vi "Dashboard Main.vi"() -> ()   [LabVIEW 2023]
uses:
  52f2dcef-b32f-41dc-9262-467f65fbdc6c.vi
  <vilib>/Rock Robotics/Network Tables/NT Write String Array.vi
  <vilib>/Rock Robotics/WPI/Dashboard/WPI_DashboardLogging Global.vi
  <vilib>/Rock Robotics/Network Tables/NT Write Boolean.vi
panel:
  in  "Camera Settings Right":T1={"Frame Rate"=30, "Compression"=30, "Size"=1, "DB Camera Config"=FALSE} {"Frame Rate" scale=1.0..30.0; "Compression" scale=100.0..-1.0; "Size" items=["640x480", "320x240", "160x120"]}
  in  "Camera Name Right":string(combo)="No Camera Selection"
  out "NT Connection":bool
  in  "Camera Settings":T1={"Frame Rate"=30, "Compression"=30, "Size"=1, "DB Camera Config"=FALSE} {"Frame Rate" scale=1.0..30.0; "Compression" scale=100.0..-1.0; "Size" items=["640x480", "320x240", "160x120"]}
  in  "Camera Name":string(combo)="No Camera Selection"
  in  "TCP":refnum<k5>
  in  "Rec Mode":enum32{"Stop", "Record", "Playback"}(radio)
  out "Robot IP":string
  out "Image Message":string="Timeout in Camera Communications"
  in  "Dashboard Tab":T2(tab)
  out "Bottom Left Flywheel":dbl
  out "Top Left Flywheel":dbl
  in  "Battery Used":string
  in  "Auto Delay?":bool
  in  "Delay Time (s)":dbl
  out "Climb 2":dbl
  in  "Aquitaine File":string
  in  "Climb Arm Reset":bool
  out "Climb 1":dbl
  out "Bottom Right Flywheel":dbl
  out "Top Right Flywheel":dbl
  in  "Shooter Hood Reset":bool
  in  "Auto Calibrate":bool=TRUE
  in  "Robot Selector":u16(ring) items=["2468 Competition", "2468 Practice"]
  in  "Manual Paths":string[](array[string])
  in  "Max Rotation":dbl=270.0
  in  "Max Translation":dbl=19.0
  in  "Deadband":dbl=0.05
  in  "Auto Selector":T3(ring)
  out "IMU":dbl(knob) scale=-180.0..180.0
  in  "Select Auto":string(combo)="Select Autonomous ..."
  out "Mode":T4(ring)=enum."Auto Disabled"
  out "Camera Perf":cluster{"Bandwidth (Mbps)":dbl, "FPS":dbl}
  out "Shooter Hood":dbl
  out "Camera Perf 2":string
  out "Auto Picture":picture
  in  "Amp Scale":dbl=0.97
  out "Shooter Hood":dbl
  out "Distance from Speaker":dbl
  out "Trap Auto Align":bool
  out "Camera Image Right":T5(plugin-control)
  out "Speaker Auto Align":bool
  out "Field Centric":bool
  out "Camera Image":T5(plugin-control)
  out "Current Shot":T6(ring)
  out "In Range?":bool
  out "Tree":string(tree)
  # "HW"
  # "HW"
  # "IMU"
  # "SWERVE"
  # "AUTONOMOUS"
  # "CONFIGS"
  # "FEEDBACK"
  # "INTAKE VIEW"
  # "SHOOTER VIEW"
  # "FIELD CENTRIC"
  # "SPEAKER AA"
  # "TRAP AA"
  # "CAN ERROR"
  # "SENSOR FAULT"
  # "GATE DRIVER"
  # "No POWER"
  # "FuLL FORWARD"
  # "FuLL REVERSE"
  # "BRUSHED BRAKE"
  # "BRUSHED COAST"
  # "BRUSHLESS BRAKE"
  # "BRUSHLESS COAST"
  # "RECOVERY MODE/OFF"
  # "https://cdn8.bigcommerce.com/s-t3eo8vwp22/product_images/uploaded_images/fault-no-12v.gif"
  # "PIGEON 2"
  # "DAMAGED HARDWARE"
  # "BOOTLOADER"
  # "CAN FAULT"
  # "ROBOT DISABLED"
  # "ROBOT ENABLED"
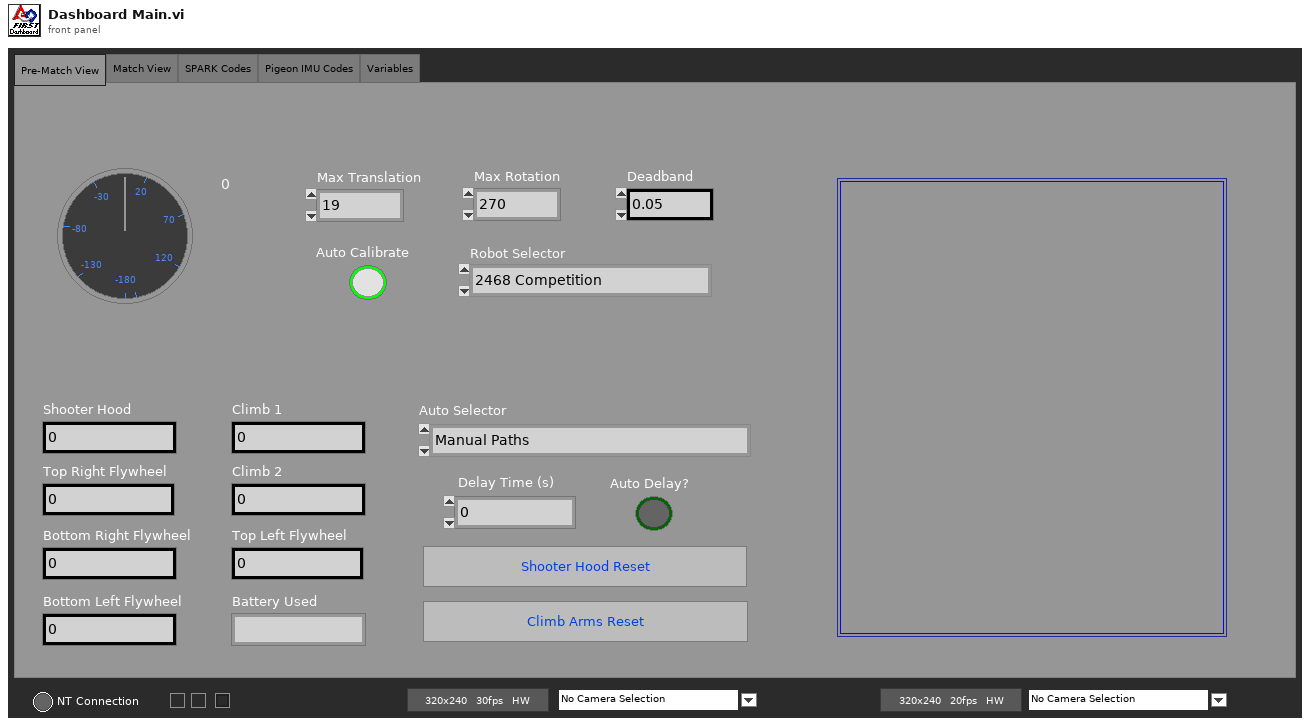
[diagram p1: front panel]
types:
  T1 = cluster{"Frame Rate":i32, "Compression":i32, "Size":u16, "DB Camera Config":bool}
  T2 = enum32{"Pre-Match View", "Match View", "SPARK Codes", "Pigeon IMU Codes", "Variables"}
  T3 = enum16{"Manual Paths", "Center - 5 Note (Line + 3rd)", "Center - 4 Note (Line + Sprint)", "Amp RED - 5 Note (1 then 3)", "Amp BLUE - 5 Note (1 then 3)", "Source RED - 3 Note (5, 4, Sprint)", "Source BLUE - 3 Note (5, 4, Sprint)", "Source RED - 3 Note (4, 5, Sprint)", "Source BLUE - 3 Note (4, 5, Sprint)", "Center - 5 Note (3, 2, 4)"}
  T4 = enum8{"Tele-Op Disabled", "Tele-Op Enabled", "Auto Disabled", "Auto Enabled", "Test Disabled", "Test Enabled", "Disconnected", "No Code", "E-Stop"}
  T5 = typedef "IMAQ Image.ctl" = refnum<image>
  T6 = enum32{"Soft Lob", "Amp", "Subwoofer", "Long Lob", "Idle", "Zero", "Trap", "Interpolation"}
  T7 = cluster{"Save Path":path, "Interval (s)":dbl, "Keep":i32}
  T8 = typedef "Image Type" = u32
  T9 = enum32{"Pre-Match View", "Match View", "SparkMax Codes", "Pigeon IMU Codes", "Variables"}
  T10 = cluster{"IDs":cluster{"RPC field ID":u16, "Unique ID":u16}, "String":string}
  T11 = cluster{"Dashboard Tab":refnum<vi>, "Rec Mode":refnum<vi>, "Tree":refnum<vi>, "Camera Perf 2":refnum<vi>, "Camera Settings":refnum<vi>, "Camera Name":refnum<vi>, "Camera Image":refnum<vi>}
  T12 = cluster{"Global Rectangle":i32[], "Contours":cluster{"Contour Type":u32, "ROI Type":u32, "Points":i32[]}[]}
  T13 = cluster{"Camera Name Right":string, string, "Saved DB Images Info":cluster{"Save Path":path, "Interval (s)":dbl, "Keep":i32}}
  T14 = cluster{"Camera Name":string, string, "Saved DB Images Info":cluster{"Save Path":path, "Interval (s)":dbl, "Keep":i32}}
  T15 = cluster{"Error Strings":string, "Disable Counts":cluster{u16, u16}, "Rail Faults":cluster{u16, u16, u16}, "Robot IP":string, "DB Mode":u8, "Event Info":cluster{"Name":string, "Type":u8, "Number":u16, "Replay":u8}}
  T16 = cluster{"Storage":cluster{"Disk Free":u64, "RAM Block":u32, "RAM free":u32}, "CPU Utilization":cluster{"CPU % ISR":sgl, "CPU % Time Crit":sgl, "CPU % Timed Str":sgl, "CPU % High":sgl, "CPU % Above":sgl, "CPU % Normal":sgl, "CPU % Low":sgl}, "CAN":cluster{"% Bus Utilization":sgl, "Bus Off Cnt":u32, "TX_FIFO Full Cnt":u32, "Receive Error Cnt":u8, "Transmit Error Cnt":u8}, "HID":cluster{"HID Outputs":u32, "Rumble Low":u16, "Rumble High":u16}[]}
  T17 = cluster{"Status bits":cluster{"Test Mode":bool, "Autonomous":bool, "Enabled":bool, "Code Start":bool, "Brownout":bool, "Reserved 2":bool, "Reserved 3":bool, "E-Stop":bool}, "Code Trace":cluster{"Disabled":bool, "TeleOp":bool, "Auto":bool, "Test":bool}, "Controller Type":enum16{"unknown", "cRIO", "roboRio"}, "Code?":enum16{"unknown", "noCode", "code"}, "Battery V":dbl}
  T18 = cluster{"Control Bits":cluster{"TestMode":bool, "Autonomous":bool, "Enabled":bool, "FMS Present":bool, bool, bool, bool, "E-Stop":bool}, "Team Station ":u8, "Countdown":sgl, "Joystick Values":cluster{"Axes":dbl[], "Buttons":bool[], "POVs":i16[]}[]}
  T19 = typedef "imagedata.ctl" = cluster{"image type":i32, "image depth":i32, "image":u8[], "mask":u8[], "colors":u32[], "Rectangle":cluster{"left":i16, "top":i16, "right":i16, "bottom":i16}}
  T20 = cluster{"Operation":enum16{"Update", "Clear"}, "Color Box":u32}[]
  T21 = cluster{"Image Size":bool, "Image Type":bool, "Pixel Value":bool, "ROI Information":bool, "Zoom Factor":bool}
  T22 = cluster{"Shift":bool, "Ctrl":bool, "Alt":bool, "Cmd":bool, "Opt":bool}
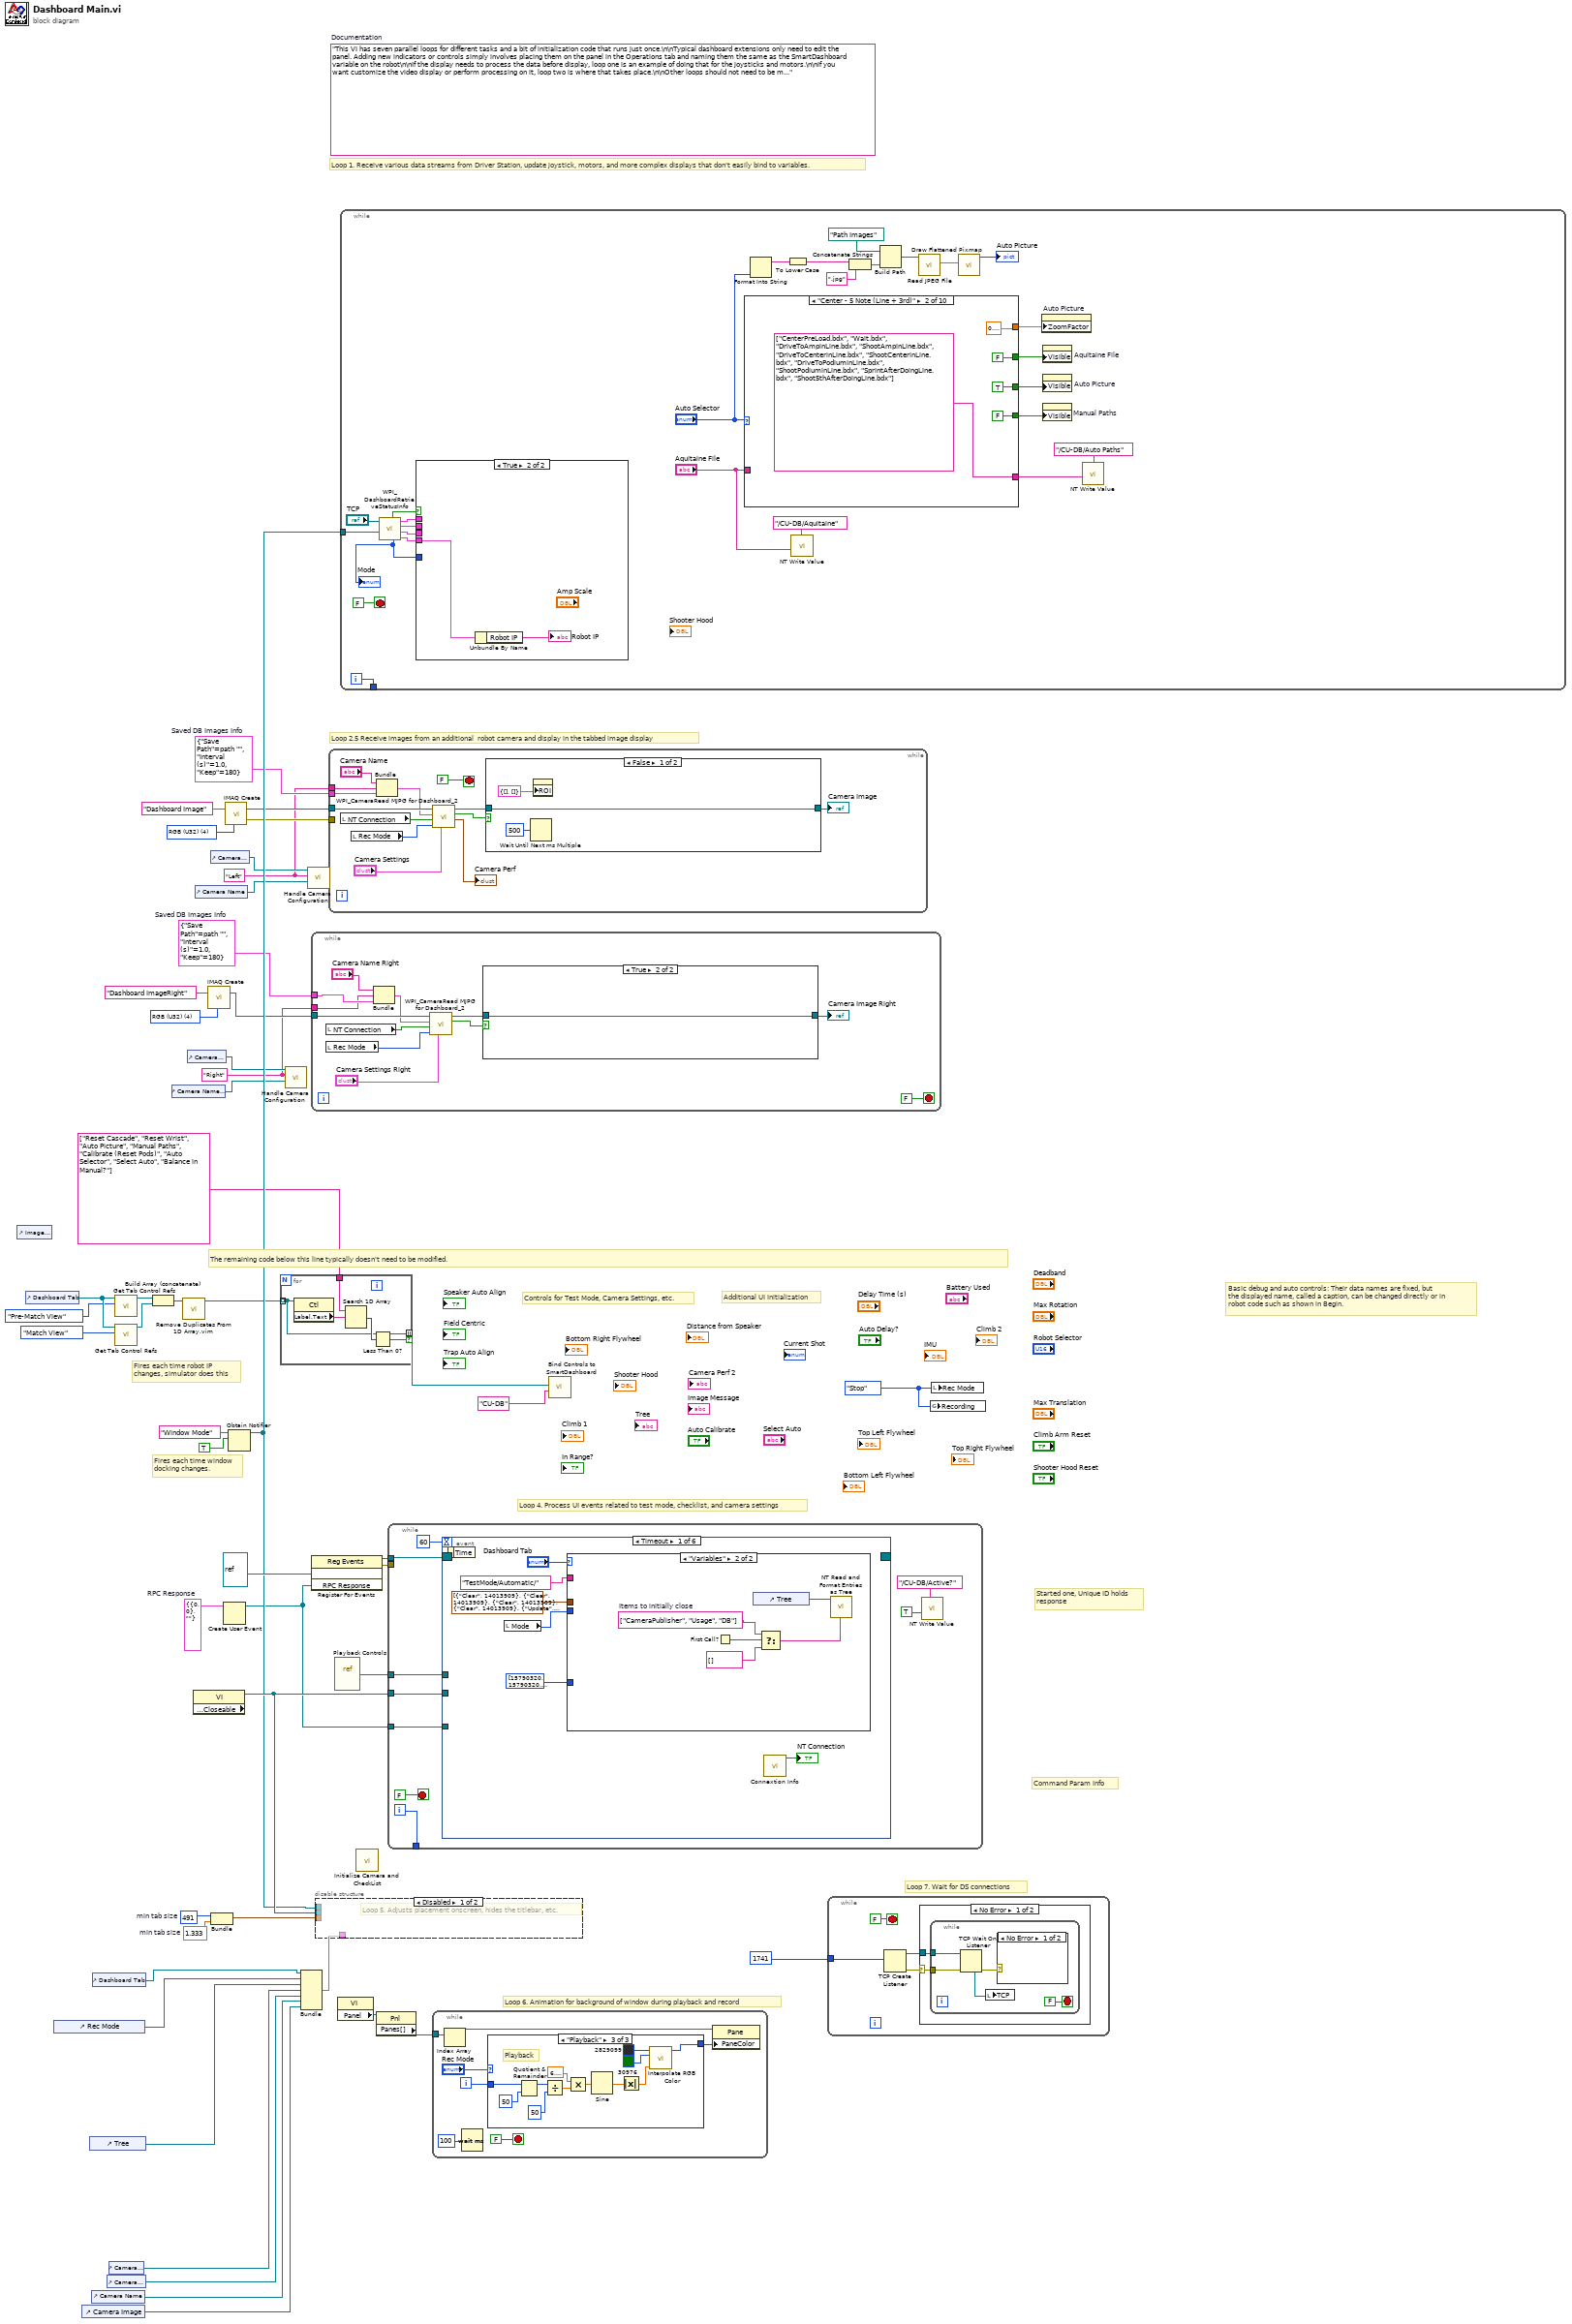
[diagram p0: block diagram]
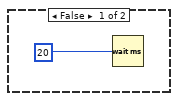
[diagram p2: hidden frame]
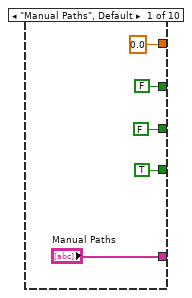
[diagram p3: hidden frame]
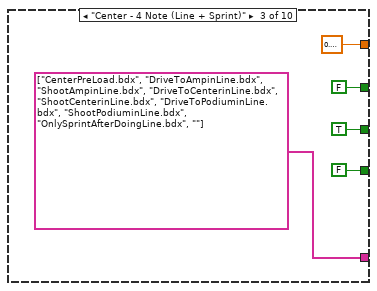
[diagram p4: hidden frame]
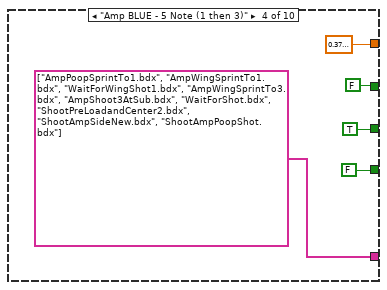
[diagram p5: hidden frame]
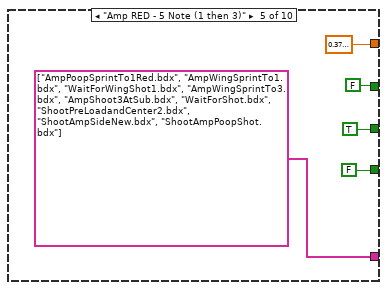
[diagram p6: hidden frame]
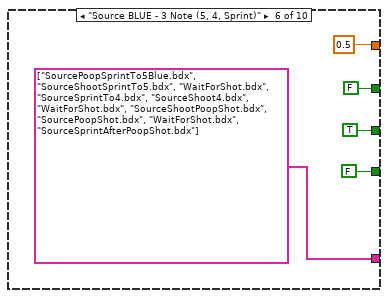
[diagram p7: hidden frame]
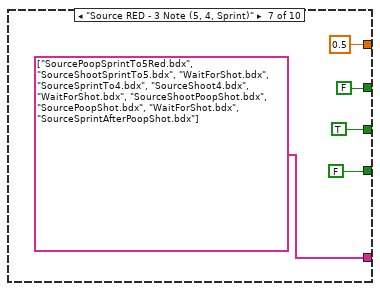
[diagram p8: hidden frame]
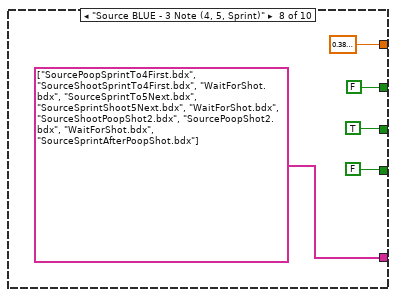
[diagram p9: hidden frame]
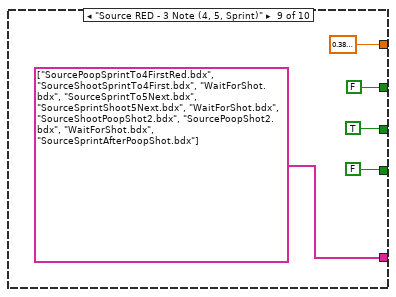
[diagram p10: hidden frame]
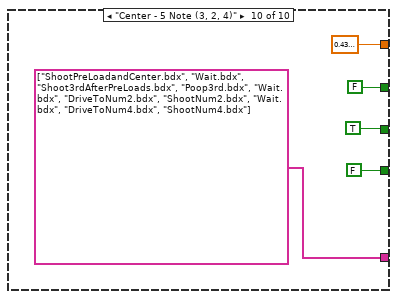
[diagram p11: hidden frame]
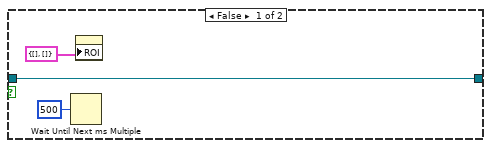
[diagram p14: hidden frame]
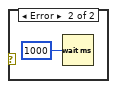
[diagram p15: hidden frame]
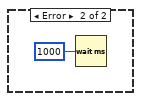
[diagram p16: hidden frame]
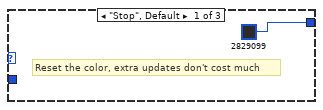
[diagram p17: hidden frame]
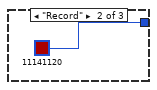
[diagram p18: hidden frame]
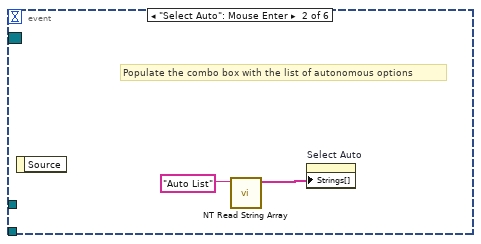
[diagram p20: hidden frame]
diagram:
  w1 = "Right"
  w6 = T7 {"Save Path"=path "", "Interval (s)"=1.0, "Keep"=180}  # Saved DB Images Info
  w8 = T8 4 items=["Grayscale (U8)", "Grayscale (I16)", "Grayscale (SGL)", "Complex (CSG)", "RGB (U32)", "HSL (U32)", "RGB (U64)"] ("Image Type")
  w24 = T7 {"Save Path"=path "", "Interval (s)"=1.0, "Keep"=180}  # Saved DB Images Info
  w5 = "Left"
  w29 = T8 4 items=["Grayscale (U8)", "Grayscale (I16)", "Grayscale (SGL)", "Complex (CSG)", "RGB (U32)", "HSL (U32)", "RGB (U64)"] ("Image Type")
  w33 = T10 {"IDs"={"RPC field ID"=0, "Unique ID"=0}, "String"=""}  # RPC Response
  w40 = 491  # min tab size
  w39 = 1.333  # min tab size
  w42 = enum32{"Stop", "Record", "Playback"}."Stop" ("Rec Mode")
  (unwired) "This VI has seven parallel loops for different tasks and a bit of initialization code that runs just once.\n\nTypical dashboard extensions only need to edit the panel. Adding new indicators or controls simply involves placing them on the panel in the Operations tab and naming them the same as the SmartDashboard variable on the robot\n\nIf the display needs to process the data before display, loop one is an example of doing that for the joysticks and motors.\n\nIf you want customize the video display or perform processing on it, loop two is where that takes place.\n\nOther loops should not need to be modified. They are pretty standard, and document the task they perform."  # Documentation
  # "Loop 2.5 Receive images from an additional  robot camera and display in the tabbed image display"
  # "Command Param Info"
  # "Started one, Unique ID holds\nresponse"
  # "Loop 7. Wait for DS connections"
  # "Basic debug and auto controls: Their data names are fixed, but\nthe displayed name, called a caption, can be changed directly or in\nrobot code such as shown in Begin."
  # "Controls for Test Mode, Camera Settings, etc."
  # "Additional UI Initialization"
  # "Loop 6. Animation for background of window during playback and record"
  # "Fires each time robot IP\nchanges, simulator does this"
  # "Fires each time window\ndocking changes."
  # "The remaining code below this line typically doesn't need to be modified."
  # "Loop 4. Process UI events related to test mode, checklist, and camera settings"
  # "Loop 1. Receive various data streams from Driver Station, update joystick, motors, and more complex displays that don't easily bind to variables."
  n1 = control-ref of="Image Message"() -> ()  [unwired: 1 out]
  n2 = control-ref of="Dashboard Tab"() -> (w22:refnum<vi>)
  n3 = control-ref of="Rec Mode"() -> (w36:refnum<vi>)
  n4 = control-ref of="Camera Image"() -> (w25:refnum<vi>)
  n5 = control-ref of="Tree"() -> (w23:refnum<vi>)
  n6 = control-ref of="Camera Name"() -> (w26:refnum<vi>)
  n7 = control-ref of="Dashboard Tab"() -> (w14:refnum<vi>)
  n8 = control-ref of="Camera Settings"() -> (w27:refnum<vi>)
  n9 = control-ref of="Camera Perf 2"() -> (w31:refnum<vi>)
  n10 = call <vilib>:"Get Tab Control Refs.vi"("Page Index"=T9."Pre-Match View" ("Dashboard Tab"), "TabControl in"=w22) -> ("ControlsOnPage"=w21:refnum<vi>[])  [unwired: 9 in]
  n11 = call <vilib>:"Get Tab Control Refs.vi"("Page Index"=T9."Match View" ("Dashboard Tab"), "TabControl in"=w22) -> ("ControlsOnPage"=w20:refnum<vi>[])  [unwired: 9 in]
  n12 = Build Array (concatenate)(w21, w20) -> (w19:refnum<vi>[])
  n13 = control-ref of="Camera Name Right"() -> (w2:refnum<vi>)
  n14 = call "Remove Duplicates From 1D Array.vim"("array"=w19) -> ("array with duplicates removed"=w16:refnum<vi>[])  [unwired: 10 in]
  n15 = control-ref of="Camera Settings Right"() -> (w3:refnum<vi>)
  n16 = property class="VI" props=["Front Panel.Closeable"]() -> (reference out=w41:refnum<vi>)  [unwired: 2 in, 2 out]
  n17 = control-ref of="Camera Name"() -> (w10:refnum<vi>)
  n18 = call "IMAQ Create"("Image Name"="Dashboard ImageRight", "Image Type"=w8) -> ("New Image"=w4:T5)  [unwired: 2 in, 2 out]
  n19 = control-ref of="Camera Settings"() -> (w11:refnum<vi>)
  n20 = Bundle("min tab size"=w40, "min tab size"=w39) -> (w38:cluster{"min tab size":i32, "min tab size":dbl})  [unwired: 1 in]
  n21 = Create User Event(user event datatype=w33) -> (user event=w32:refnum<user-event>)  [unwired: 1 in, 1 out]
  n22 = call "IMAQ Create"("Image Name"="Dashboard Image", "Image Type"=w29) -> ("New Image"=w9:T5, "error out"=w28:errorcluster)  [unwired: 2 in, 1 out]
  n23 = Obtain Notifier(name (unnamed)="Window Mode", notification data type=TRUE) -> (notifier out=w35:refnum<notifier>)  [unwired: 2 in, 2 out]
  n24 = for {
    tunnel: string[] ["Reset Cascade", "Reset Wrist", "Auto Picture", "Manual Paths", "Calibrate (Reset Pods)", "Auto Selector", "Select Auto", "Balance in Manual?"] -> [w56]
    tunnel: w16 -> [w53] mode=indexing
    tunnel: [w53] -> w15 mode=indexing if=w52
    n25 = property class="Ctl"(reference=w53) -> ("Label.Text"=w55:string)  [unwired: 1 in, 2 out]
    n26 = Search 1D Array(1D array=w56, element=w55) -> (index of element=w54:i32)  [unwired: 1 in]
    n27 = Less Than 0?(x=w54) -> (x < 0?=w52:bool)
  }
  n28 = call "Handle Camera Configuration.vi"("CameraNameRef"=w2, "Display Name"=w1, "ClusterRef"=w3) -> ()  [unwired: 9 in]
  n29 = Bundle("Dashboard Tab"=w14, "Rec Mode"=w36, "Tree"=w23, "Camera Perf 2"=w31, "Camera Settings"=w27, "Camera Name"=w26, "Camera Image"=w25) -> (w37:T11)  [unwired: 1 in]
  n30 = call "Handle Camera Configuration.vi"("CameraNameRef"=w10, "Display Name"=w5, "ClusterRef"=w11) -> ()  [unwired: 9 in]
  n31 = while {
    tunnel: w6 -> [w61]
    tunnel: w4 -> [w64]
    tunnel: w1 -> [w58]
    stop <- FALSE stop-if-true
    n32 = local read "NT Connection"() -> (w63:bool)
    n33 = local read "Rec Mode"() -> (w62:enum32{"Stop", "Record", "Playback"})
    n34 = Bundle("Camera Name Right"="Camera Name Right", w58, "Saved DB Images Info"=w61) -> (w57:T13)  [unwired: 1 in]
    n35 = call <vilib>:"WPI_CameraRead MJPG for Dashboard_2.vi"("Camera Settings"="Camera Settings Right", "Rec Mode"=w62, "NT Connection"=w63, "Capture Info"=w57, "Image in"=w64) -> ("Active"=w66:bool, "Image\\ out"=w67:T5)  [unwired: 4 in, 1 out]
    n36 = case shown="True" w66 {
      tunnel: w67 -> [w70 w72]
      tunnel: [w70 w72] -> w68
      frame False {
        n37 = Wait Until Next ms Multiple(millisecond multiple=u32 500) -> ()  [unwired: 1 out]
        n38 = property on="Camera Image" class="ImageControl"("ROI"=T12 {"Global Rectangle"=[], "Contours"=[]}) -> ()  [unwired: 2 in, 2 out]
      }
      frame True {
      }
    }
    "Camera Image Right" <- w68
  }
  n39 = register-events(refnum<vi> refnum, w32) -> (reference out=w45:refnum<event-registration>, error out=w44:errorcluster)  [unwired: 2 in]
  n40 = disable-structure shown="Disabled" {
    disable-tunnel: w41 -> [_ _]
    disable-tunnel: w38 -> [_ _]
    disable-tunnel: w37 -> [_ _]
    disable-tunnel: w35 -> [_ _]
    frame Disabled {
      # "Loop 5. Adjusts placement onscreen, hides the titlebar, etc."
    }
    frame Enabled {
    }
  }
  n41 = while {
    tunnel: w9 -> [w85]
    tunnel: w28 -> [_]
    tunnel: w24 -> [w74]
    tunnel: w5 -> [w76]
    stop <- FALSE stop-if-true
    n42 = local read "NT Connection"() -> (w75:bool)
    n43 = local read "Rec Mode"() -> (w73:enum32{"Stop", "Record", "Playback"})
    n44 = Bundle("Camera Name"="Camera Name", w76, "Saved DB Images Info"=w74) -> (w79:T14)  [unwired: 1 in]
    n45 = call <vilib>:"WPI_CameraRead MJPG for Dashboard_2.vi"("Camera Settings"="Camera Settings", "Rec Mode"=w73, "NT Connection"=w75, "Capture Info"=w79, "Image in"=w85) -> ("perf info"=→"Camera Perf":cluster{"Bandwidth (Mbps)":dbl, "fps":dbl}, "Active"=w81:bool, "Image\\ out"=w83:T5)  [unwired: 4 in]
    n46 = case shown="False" w81 {
      tunnel: w83 -> [w87 w89]
      tunnel: [w87 w89] -> w80
      frame False {
        n47 = Wait Until Next ms Multiple(millisecond multiple=u32 500) -> ()  [unwired: 1 out]
        n48 = property on="Camera Image" class="ImageControl"("ROI"=T12 {"Global Rectangle"=[], "Contours"=[]}) -> ()  [unwired: 2 in, 2 out]
      }
      frame True {
      }
    }
    "Camera Image" <- w80
  }
  n49 = vi-ref "Playback Controls.vi"() -> (w46:refnum<vi>)
  n50 = property class="VI"() -> ("Panel"=w48:refnum<vi>)  [unwired: 2 in, 2 out]
  n51 = while {
    tunnel: [w115] -> _
    tunnel: w35 -> [w108]
    i -> [w115]
    stop <- FALSE stop-if-true
    n52 = call <vilib>:"WPI_DashboardRetrieveStatusInfo.vi"("Window Mode Notifier"=w108, "TCP Cnx"="TCP") -> ("Power and Errors"=w110:T15, "Robot Metrics"=w113:T16, "Status Info"=w114:T17, "Control Info"=w111:T18, "Robot Mode"=w91:T4, "Process?"=w112:bool)  [unwired: 4 in]
    "Mode" <- w91
    n53 = case shown="True" w112 {
      tunnel: w114 -> [_ _]
      tunnel: w113 -> [_ _]
      tunnel: w111 -> [_ _]
      tunnel: w110 -> [_ w119]
      tunnel: w91 -> [_ _]
      frame False {
        n54 = Wait (ms)(milliseconds to wait=u32 20) -> ()  [unwired: 1 out]
      }
      frame True {
        n55 = Unbundle By Name(w119) -> ("Robot IP"=→"Robot IP":string)
      }
    }
    n56 = case shown="\"Center - 5 Note (Line + 3rd)\"" "Auto Selector" {
      tunnel: ["Manual Paths" string[] ["CenterPreLoad.bdx", "Wait.bdx", "DriveToAmpinLine.bdx", "ShootAmpinLine.bdx", "DriveToCenterinLine.bdx", "ShootCenterinLine.bdx", "DriveToPodiuminLine.bdx", "ShootPodiuminLine.bdx", "SprintAfterDoingLine.bdx", "Shoot5thAfterDoingLine.bdx"] ("Manual Paths") string[] ["CenterPreLoad.bdx", "DriveToAmpinLine.bdx", "ShootAmpinLine.bdx", "DriveToCenterinLine.bdx", "ShootCenterinLine.bdx", "DriveToPodiuminLine.bdx", "ShootPodiuminLine.bdx", "OnlySprintAfterDoingLine.bdx", ""] ("Manual Paths") string[] ["AmpPoopSprintTo1.bdx", "AmpWingSprintTo1.bdx", "WaitForWingShot1.bdx", "AmpWingSprintTo3.bdx", "AmpShoot3AtSub.bdx", "WaitForShot.bdx", "ShootPreLoadandCenter2.bdx", "ShootAmpSideNew.bdx", "ShootAmpPoopShot.bdx"] ("Manual Paths") string[] ["AmpPoopSprintTo1Red.bdx", "AmpWingSprintTo1.bdx", "WaitForWingShot1.bdx", "AmpWingSprintTo3.bdx", "AmpShoot3AtSub.bdx", "WaitForShot.bdx", "ShootPreLoadandCenter2.bdx", "ShootAmpSideNew.bdx", "ShootAmpPoopShot.bdx"] ("Manual Paths") string[] ["SourcePoopSprintTo5Blue.bdx", "SourceShootSprintTo5.bdx", "WaitForShot.bdx", "SourceSprintTo4.bdx", "SourceShoot4.bdx", "WaitForShot.bdx", "SourceShootPoopShot.bdx", "SourcePoopShot.bdx", "WaitForShot.bdx", "SourceSprintAfterPoopShot.bdx"] ("Manual Paths") string[] ["SourcePoopSprintTo5Red.bdx", "SourceShootSprintTo5.bdx", "WaitForShot.bdx", "SourceSprintTo4.bdx", "SourceShoot4.bdx", "WaitForShot.bdx", "SourceShootPoopShot.bdx", "SourcePoopShot.bdx", "WaitForShot.bdx", "SourceSprintAfterPoopShot.bdx"] ("Manual Paths") string[] ["SourcePoopSprintTo4First.bdx", "SourceShootSprintTo4First.bdx", "WaitForShot.bdx", "SourceSprintTo5Next.bdx", "SourceSprintShoot5Next.bdx", "WaitForShot.bdx", "SourceShootPoopShot2.bdx", "SourcePoopShot2.bdx", "WaitForShot.bdx", "SourceSprintAfterPoopShot.bdx"] ("Manual Paths") string[] ["SourcePoopSprintTo4FirstRed.bdx", "SourceShootSprintTo4First.bdx", "WaitForShot.bdx", "SourceSprintTo5Next.bdx", "SourceSprintShoot5Next.bdx", "WaitForShot.bdx", "SourceShootPoopShot2.bdx", "SourcePoopShot2.bdx", "WaitForShot.bdx", "SourceSprintAfterPoopShot.bdx"] ("Manual Paths") string[] ["ShootPreLoadandCenter.bdx", "Wait.bdx", "Shoot3rdAfterPreLoads.bdx", "Poop3rd.bdx", "Wait.bdx", "DriveToNum2.bdx", "ShootNum2.bdx", "Wait.bdx", "DriveToNum4.bdx", "ShootNum4.bdx"] ("Manual Paths")] -> w107
      tunnel: [FALSE ("Visible") TRUE ("Visible") TRUE ("Visible") TRUE ("Visible") TRUE ("Visible") TRUE ("Visible") TRUE ("Visible") TRUE ("Visible") TRUE ("Visible") TRUE ("Visible")] -> w106
      tunnel: [TRUE ("Visible") FALSE ("Visible") FALSE ("Visible") FALSE ("Visible") FALSE ("Visible") FALSE ("Visible") FALSE ("Visible") FALSE ("Visible") FALSE ("Visible") FALSE ("Visible")] -> w93
      tunnel: [FALSE ("Visible") FALSE ("Visible") FALSE ("Visible") FALSE ("Visible") FALSE ("Visible") FALSE ("Visible") FALSE ("Visible") FALSE ("Visible") FALSE ("Visible") FALSE ("Visible")] -> w103
      tunnel: "Aquitaine File" -> [_ _ _ _ _ _ _ _ _ _]
      tunnel: [sgl 0.0 ("Zoom Factor") sgl 0.4 ("Zoom Factor") sgl 0.4 ("Zoom Factor") sgl 0.37 ("Zoom Factor") sgl 0.37 ("Zoom Factor") sgl 0.5 ("Zoom Factor") sgl 0.5 ("Zoom Factor") sgl 0.39 ("Zoom Factor") sgl 0.39 ("Zoom Factor") sgl 0.44 ("Zoom Factor")] -> w90
      frame "Manual Paths", Default {
      }
      frame "Center - 5 Note (Line + 3rd)" {
      }
      frame "Center - 4 Note (Line + Sprint)" {
      }
      frame "Amp BLUE - 5 Note (1 then 3)" {
      }
      frame "Amp RED - 5 Note (1 then 3)" {
      }
      frame "Source BLUE - 3 Note (5, 4, Sprint)" {
      }
      frame "Source RED - 3 Note (5, 4, Sprint)" {
      }
      frame "Source BLUE - 3 Note (4, 5, Sprint)" {
      }
      frame "Source RED - 3 Note (4, 5, Sprint)" {
      }
      frame "Center - 5 Note (3, 2, 4)" {
      }
    }
    n57 = Format Into String("Auto Selector") -> (resulting string=w97:string)  [unwired: 3 in, 1 out]
    n58 = To Lower Case(string=w97) -> (all lower case string=w98:string)
    n59 = call-poly <vilib>:"NT Write Value.vi"("value"="Aquitaine File", "name"="/CU-DB/Aquitaine") -> ()  [unwired: 9 in, 1 out]
    n60 = Concatenate Strings(w98, ".jpg" ("string")) -> (w99:string)
    n61 = Build Path(base path=path "Path Images", name or relative path=w99) -> (appended path=w102:path)
    n62 = call <vilib>:"Read JPEG File.vi"("path to JPEG file"=w102) -> ("image data"=w101:T19)  [unwired: 8 in, 2 out]
    n63 = call <vilib>:"Draw Flattened Pixmap.vi"("image data"=w101) -> ("new picture"=→"Auto Picture":picture)  [unwired: 8 in]
    n64 = property on="Auto Picture" class="Pict"("ZoomFactor"=w90) -> ()  [unwired: 2 in, 2 out]
    n65 = property on="Aquitaine File" class="Str"("Visible"=w103) -> ()  [unwired: 2 in, 2 out]
    n66 = property on="Auto Picture" class="Pict"("Visible"=w106) -> ()  [unwired: 2 in, 2 out]
    n67 = property on="Manual Paths" class="Arr (strict)"("Visible"=w93) -> ()  [unwired: 2 in, 2 out]
    n68 = call-poly <vilib>:"NT Write Value.vi"("value"=w107, "name"="/CU-DB/Auto Paths") -> ()  [unwired: 9 in, 1 out]
  }
  n69 = call "Initialize Camera and CheckList.vi"() -> ()  [unwired: 12 in]
  n70 = property class="Pnl"(reference=w48) -> ("Panes[]"=w49:refnum<vi>[])  [unwired: 1 in, 2 out]
  n71 = while {
    tunnel: [w176] -> _
    tunnel: w46 -> [w175]
    tunnel: w45 -> [w174]
    tunnel: w44 -> [_]
    tunnel: w41 -> [w173]
    tunnel: w32 -> [w172]
    i -> [w176]
    stop <- FALSE stop-if-true
    n72 = event shown="[0] Timeout" {
      selector: w174 -> [_ _ _ _ _ _]
      dyn-events: [_ _ _ w200 _ _] -> _
      timeout: u32 60 ("milliseconds to wait") -> [_ _ _ _ _ _]
      tunnel: w175 -> [_ _ _ w202 w217 _]
      tunnel: w173 -> [_ _ _ w198 _ _]
      tunnel: w172 -> [_ _ _ w196 _ _]
      event Timeout {
        n73 = event-data() -> ()  [unwired: 1 in, 1 out]
        n74 = local read "Mode"() -> (w181:T4)
        n75 = case shown="\"Variables\"" "Dashboard Tab" {
          tunnel: "TestMode/Automatic/" ("Name Pattern") -> [_ _]
          tunnel: T20 [{"Operation"=enum."Clear", "Color Box"=14013909}, {"Operation"=enum."Clear", "Color Box"=14013909}, {"Operation"=enum."Clear", "Color Box"=14013909}, {"Operation"=enum."Clear", "Color Box"=14013909}, {"Operation"=enum."Update", "Color Box"=14013909}, {"Operation"=enum."Update", "Color Box"=16777215}, {"Operation"=enum."Clear", "Color Box"=14013909}, {"Operation"=enum."Clear", "Color Box"=14013909}, {"Operation"=enum."Clear", "Color Box"=14013909}] -> [_ _]
          tunnel: w181 -> [_ _]
          tunnel: u32[] [15790320, 15790320, 15790320, 15790320, 16777215, 16777215, 15790320, 15790320, 15790320] -> [_ _]
          frame Default {
          }
          frame "Variables" {
            w187 = string[] ["CameraPublisher", "Usage", "DB"]  # Items to initially close
            n76 = First Call?() -> (First Call?: T/F=w188:bool)
            n77 = control-ref of="Tree"() -> (w189:refnum<vi>)
            n78 = Select(t=w187, s=w188, f=string[] []) -> (s? t:f=w185:string[])
            n79 = call <vilib>:"NT Read and Format Entries as Tree.vi"("Tags to  Close"=w185, "Tree Refnum"=w189) -> ()  [unwired: 8 in, 2 out]
          }
        }
        n80 = call <vilib>:"Connextion Info.vi"() -> ("Connected"=→"NT Connection":bool)  [unwired: 10 in, 1 out]
      }
      event "Select Auto": Mouse Enter {
        # "Populate the combo box with the list of autonomous options"
        n81 = event-data() -> ()  [unwired: 1 in, 1 out]
        n82 = call <vilib>:"NT Read String Array.vi"("name"="Auto List" ("Name")) -> ("value"=w190:string[])  [unwired: 8 in, 2 out]
        n83 = property on="Select Auto" class="CmbBox"("Strings[]"=w190) -> ()  [unwired: 2 in, 2 out]
      }
      event "Select Auto": Value Change {
        # "User modified the Auto Selection. Write to NT variable so robot knows."
        n84 = event-data() -> ("NewVal"=w192:string)  [unwired: 1 in]
        n85 = call <vilib>:"NT Write String.vi"("value"=w192, "name"="Auto Selector" ("Name")) -> ()  [unwired: 9 in, 1 out]
      }
      event "Rec Mode": Value Change {
        # "Update globals for recording mode and path to read log from.\nClear when logging and let NetworkTables set path for vision to\nuse."
        n86 = event-data() -> ("NewVal"=w203:enum32{"Stop", "Record", "Playback"})  [unwired: 1 in]
        n87 = global write "WPI_DashboardLogging Global.vi" "Logging Filename"(path "") -> ()
        n88 = global write "WPI_DashboardLogging Global.vi" "Recording"(w203) -> ()
        n89 = case shown="\"Playback\"" w203 {
          tunnel: w202 -> [_ w205 w214]
          tunnel: [_ _ w213] -> w200
          tunnel: [_ _ w212] -> _
          tunnel: w198 -> [_ _ w210]
          tunnel: cluster{i32, i32} {-250, 170} -> [_ _ w209]
          tunnel: [_ _ T21 {"Image Size"=TRUE, "Image Type"=TRUE, "Pixel Value"=TRUE, "ROI Information"=TRUE, "Zoom Factor"=FALSE} ("Image Information Shown:All Elements")] -> w194
          tunnel: [_ _ TRUE ("Zoom Factor")] -> w195
          tunnel: w196 -> [_ _ w206]
          frame Default {
          }
          frame "Stop", "Record" {
            # "Place Window too"
            n90 = invoke class="VI" method="FP.Close"(reference=w205) -> (reference out=w204:refnum<vi>)  [unwired: 2 in, 2 out]
            n91 = invoke class="VI" method="Abort VI"(reference=w204) -> ()  [unwired: 2 in, 3 out]
          }
          frame "Playback" {
            n92 = call "Open Playback Panel.vi"("Offset"=w209, "DB VI Ref"=w210, "Playback in"=w214) -> ("Playback out"=w211:refnum<vi>)  [unwired: 8 in]
            n93 = register-events(w211, w206) -> (reference out=w213:refnum<event-registration>, error out=w212:errorcluster)  [unwired: 2 in]
          }
        }
        n94 = property on="Camera Image" class="ImageControl"("Image Information Shown"=w194, "Image Information Visible"=w195) -> ()  [unwired: 2 in, 2 out]
        n95 = call <vilib>:"WPI_DashboardNT Log FieldName Cache.vi"("Operation"=enum16{"Lookup/Add", "Index", "Clear"}."Clear") -> ()  [unwired: 8 in, 3 out]
      }
      event Panel Close {
        # "Abort playback window and ourself"
        n96 = event-data() -> ()  [unwired: 1 in, 4 out]
        n97 = invoke class="VI" method="FP.Close"(reference=w217) -> (reference out=w216:refnum<vi>)  [unwired: 2 in, 2 out]
        n98 = invoke class="VI" method="Abort VI"(reference=w216) -> (error out=w215:errorcluster)  [unwired: 2 in, 2 out]
        n99 = invoke class="VI" method="Abort VI"(error in=w215) -> ()  [unwired: 2 in, 3 out]
      }
      event "Tree": Double Click {
        n100 = event-data() -> ("PlatMods"=w223:T22, "Tag"=w220:string)  [unwired: 1 in]
        n101 = Unbundle(w223) -> ("Shift"=w222:bool)  [unwired: 4 out]
        n102 = String Subset(string=w220, length (rest)=1 ("length (rest)")) -> (substring=w219:string)  [unwired: 1 in]
        n103 = Not(x=w222) -> (.not. x?=w221:bool)
        n104 = case shown="\"/\"" w219 {
          tunnel: w220 -> [_ w225]
          tunnel: w221 -> [_ w224]
          frame Default {
          }
          frame "/" {
            n105 = call <vilib>:"NT Update Persistence.vi"("Persistence"=w224, "Name"=w225) -> ()  [unwired: 9 in, 1 out]
          }
        }
      }
    }
    n106 = call-poly <vilib>:"NT Write Value.vi"("value"=TRUE ("Boolean"), "name"="/CU-DB/Active?" ("Name")) -> ()  [unwired: 9 in, 1 out]
  }
  n107 = Index Array(array=w49) -> (element=w47:refnum<vi>)  [unwired: 1 in]
  n108 = while {
    tunnel: w47 -> [w227]
    i -> [w230]
    stop <- FALSE stop-if-true
    n109 = Wait (ms)(milliseconds to wait=u32 100) -> ()  [unwired: 1 out]
    n110 = case shown="\"Playback\"" "Rec Mode" {
      tunnel: w230 -> [_ _ w245]
      tunnel: [u32 2829099 ("Base Color") u32 11141120 ("Target Color") w234] -> w226
      frame "Stop", Default {
        # "Reset the color, extra updates don't cost much"
      }
      frame "Record" {
      }
      frame "Playback" {
        # "Playback"
        n111 = Quotient & Remainder(x=w245, y=u32 50 ("milliseconds to wait")) -> (x-y*floor(x/y)=w241:u32)  [unwired: 1 out]
        n112 = Divide(x=w241, y=u32 50 ("milliseconds to wait")) -> (x/y=w238:dbl)
        n113 = Multiply(x=6.283185307179586, y=w238) -> (x*y=w243:dbl)
        n114 = Sine(x=w243) -> (sin(x)=w242:dbl)
        n115 = Absolute Value(x=w242) -> (abs(x)=w235:dbl)
        n116 = call "Interpolate RGB Color.vi"("Proportion"=w235, "Target Color"=u32 30976, "Base Color"=u32 2829099) -> ("Result Color"=w234:u32)  [unwired: 8 in]
      }
    }
    n117 = property class="Pane"(reference=w227, "PaneColor"=w226) -> ()  [unwired: 1 in, 2 out]
  }
  n118 = call <vilib>:"Bind Controls to SmartDashboard.vi"("Path Prefix"="CU-DB", "Bound Control Refs"=w15) -> ()  [unwired: 10 in]
  n119 = while {
    tunnel: u16 1741 ("timeout ms (25000)") -> [w247]
    stop <- FALSE stop-if-true
    n120 = TCP Create Listener(10:w247) -> (0:w246:errorcluster, 3:w248:refnum<k5>)  [unwired: 4 in, 1 out]
    n121 = case shown="No Error" w246 {
      selector: w246 -> [w250 _]
      tunnel: w248 -> [w251 _]
      frame No Error {
        n122 = while {
          tunnel: w251 -> [w254]
          tunnel: w250 -> [w253]
          stop <- FALSE stop-if-true
          n123 = TCP Wait On Listener(8:w253, 11:w254) -> (0:w255:errorcluster, 4:w256:refnum<k5>)  [unwired: 2 in, 3 out]
          n124 = local write "TCP"(w256) -> ()
          n125 = case shown="No Error" w255 {
            frame No Error {
            }
            frame Error {
              n126 = Wait (ms)(milliseconds to wait=u32 1000) -> ()  [unwired: 1 out]
            }
          }
        }
      }
      frame Error {
        n127 = Wait (ms)(milliseconds to wait=u32 1000) -> ()  [unwired: 1 out]
      }
    }
  }
  n128 = global write "WPI_DashboardLogging Global.vi" "Recording"(w42) -> ()
  n129 = local write "Rec Mode"(w42) -> ()
